vi "pd_signals_delay_trigger.vi"() -> ()   [LabVIEW 2010]
uses:
  <vilib>/Utility/error.llb/DialogType.ctl
  <vilib>/express/express arith-compare/Formula/XNode/ExpressFormulaBlockNode.xnode
  <vilib>/DAQmx/read.llb/DAQmx Read.vi
  <vilib>/DAQmx/create/channels.llb/DAQmx Create Channel (AI-Voltage-Basic).vi
  <vilib>/DAQmx/configure/timing.llb/DAQmx Timing (Sample Clock).vi
  <vilib>/DAQmx/configure/trigger.llb/DAQmx Start Trigger (Digital Edge).vi
  <vilib>/daqmx/miscellaneous.llb/DAQmx Fill In Error Info.vi
  <vilib>/express/express shared/transition.llb/Dynamic To Waveform Array.vi
  <vilib>/express/express shared/transition.llb/Waveform Array To Dynamic.vi
  <vilib>/express/express arith-compare/Formula/Block/exnFormulaBlock how many pts in the wave.vi
  <vilib>/express/express shared/ex_Modify Signal Name.vi
panel:
  in  "physical channels":tag="Dev1/ai0"
  out "Signal":waveform(dbl)[](graph)
  in  "Ring":u16(ring)=1 items=["Ref", "OA", "CA"]
  in  "Samples/channel":dbl=80.0
  in  "stop 2":bool
  out "Trigger delay":dbl format="%#_6e"
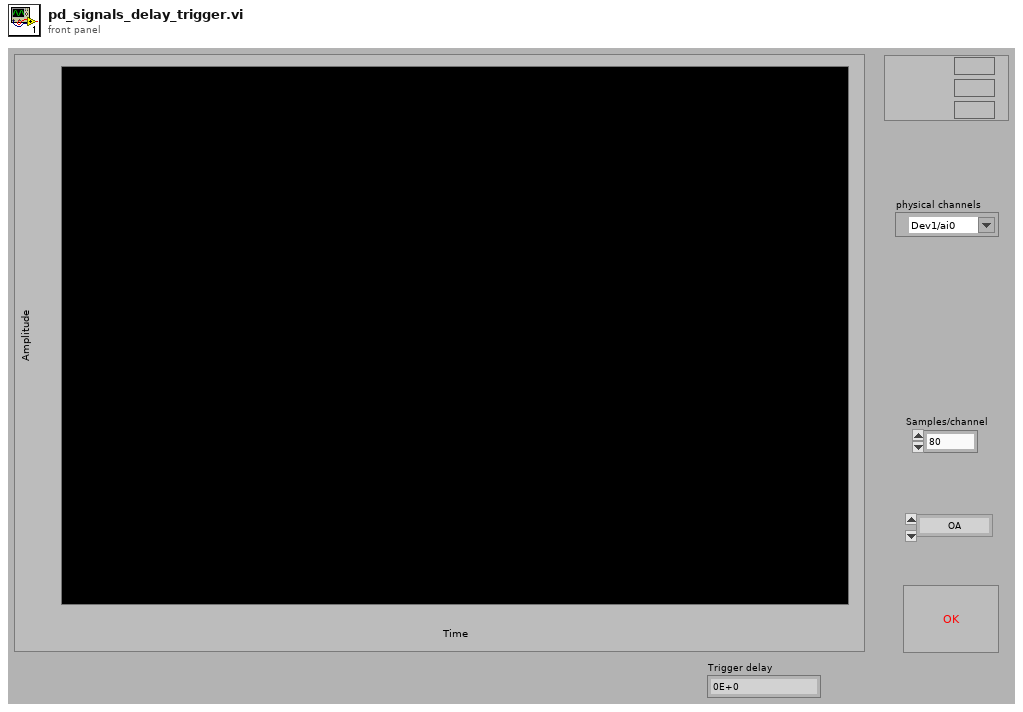
[diagram p1: front panel]
types:
  T1 = typedef "DialogType.ctl" = u16
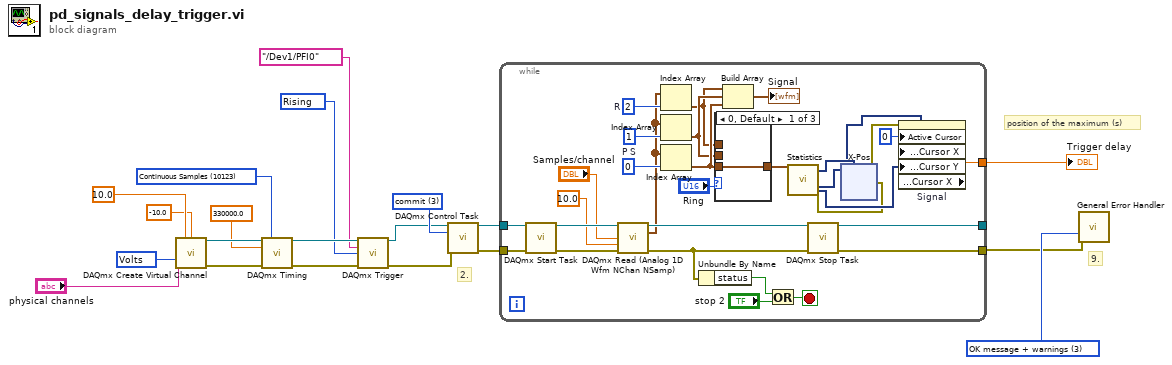
[diagram p0: block diagram]
diagram:
  w11 = 10280 items=["Rising"=10280, "Falling"=10171] ("edge")
  w9 = T1 3 items=["no dialog", "OK message", "continue or stop message", "OK message + warnings", "continue/stop + warnings"] ("type of dialog (OK msg:1)")
  w10 = 3 items=["verify"=2, "reserve"=4, "commit"=3, "unreserve"=5, "abort"=6] ("action")
  w13 = 10123 items=["Finite Samples"=10178, "Continuous Samples"=10123, "Hardware Timed Single Point"=12522] ("sample mode")
  w17 = 10348 items=["Volts"=10348, "From Custom Scale"=10065] ("units")
  # "position of the maximum (s)"
  # "9."
  # "2."
  n1 = call-poly <vilib>:"DAQmx Create Virtual Channel.vi"("maximum value"=10.0, "minimum value"=-10.0, "physical channels"="physical channels", "units"=w17) -> ("task out"=w16:refnum<k21>, "error out"=w7:errorcluster)  [unwired: 10 in]
  n2 = call-poly <vilib>:"DAQmx Timing.vi"("task/channels in"=w16, "sample mode"=w13, "rate"=330000.0, "error in"=w7) -> ("task out"=w15:refnum<k21>, "error out"=w8:errorcluster)  [unwired: 10 in]
  n3 = call-poly <vilib>:"DAQmx Trigger.vi"("task/channels in"=w15, "source"=tag "/Dev1/PFI0", "edge"=w11, "error in"=w8) -> ("task out"=w6:refnum<k21>, "error out"=w5:errorcluster)  [unwired: 10 in]
  n4 = call <vilib>:"DAQmx Control Task.vi"("task/channels in"=w6, "action"=w10, "error in"=w5) -> ("task out"=w4:refnum<k21>, "error out"=w3:errorcluster)  [unwired: 11 in]
  n5 = while {
    tunnel: w4 -> [w51]
    tunnel: w3 -> [w50]
    tunnel: [w49] -> w1
    tunnel: [w27] -> _
    tunnel: [w26] -> w2
    stop <- w22 stop-if-true
    w42 = 0  # P
    w43 = 1  # S
    w44 = 2  # R
    n6 = call <vilib>:"DAQmx Start Task.vi"("task/channels in"=w51, "error in"=w50) -> ("task out"=w48:refnum<k21>, "error out"=w47:errorcluster)  [unwired: 12 in]
    n7 = call-poly <vilib>:"DAQmx Read (Analog 1D Wfm NChan NSamp).vi"("task/channels in"=w48, "number of samples per channel"="Samples/channel", "timeout"=10.0, "error in"=w47) -> ("task out"=w46:refnum<k21>, "data"=w41:waveform(dbl)[], "error out"=w24:errorcluster)  [unwired: 9 in]
    n8 = Index Array(array=w41, index=w44) -> (element=w33:waveform(dbl))
    n9 = Index Array(array=w41, index=w43) -> (element=w34:waveform(dbl))
    n10 = Index Array(array=w41, index=w42) -> (element=w36:waveform(dbl))
    n11 = Unbundle By Name(w24) -> ("status"=w25:bool)
    n12 = case shown="0, Default" "Ring" {
      tunnel: w36 -> [w191 _ _]
      tunnel: [w191 w192 w193] -> w35
      tunnel: w34 -> [_ w192 _]
      tunnel: w33 -> [_ _ w193]
      frame 0, Default {
      }
      frame 1 {
      }
      frame 2 {
      }
    }
    n13 = Build Array(w33, w34, w36) -> (→"Signal":waveform(dbl)[])
    n14 = Or(x=w25, y="stop 2") -> (x .or. y?=w22:bool)
    n15 = call "Statistics"("Signals"=w35) -> ("First Time"=w38:dynamicdata, "Time of Maximum"=w39:dynamicdata, "Maximum"=w37:dynamicdata, "error out"=w32:errorcluster)  [unwired: 21 in, 2 out]
    n16 = call <vilib>:"DAQmx Stop Task.vi"("task/channels in"=w46, "error in"=w24) -> ("task out"=w27:refnum<k21>, "error out"=w26:errorcluster)  [unwired: 12 in]
    n17 = xnode "X-Pos"("TimeMax"=w39, "1stTime"=w38, "error in (no error)"=w32) -> ("Result"=w28:dynamicdata, "error out"=w31:errorcluster)
    n18 = property on="Signal" class="WFGraph (strict)"(error in=w31, "Active Cursor"=u32 0, "Cursor.Cursor Position:Cursor X"=w28, "Cursor.Cursor Position:Cursor Y"=w37) -> ("Cursor.Cursor Position:Cursor X"=w49:dbl)  [unwired: 1 in, 2 out]
  }
  "Trigger delay" <- w1
  n19 = call <vilib>:"General Error Handler.vi"("type of dialog (OK msg:1)"=w9, "error in (no error)"=w2) -> ()  [unwired: 9 in, 5 out]
